vi "lockin - replace AO Sweep Indicator.vi"(8 "error in (no error)":errorcluster, 10 "Channels: AO.Sweep?":bool[](array[boolean]), 11 "LockinDAQ":refnum<class "LockinDAQ.lvclass">) -> (0 "error out":errorcluster, 3 "LockinDAQ out":refnum<class "LockinDAQ.lvclass">)   [LabVIEW 2019, in "LockinDAQ.lvclass"]
uses:
  LockinDAQ.lvclass
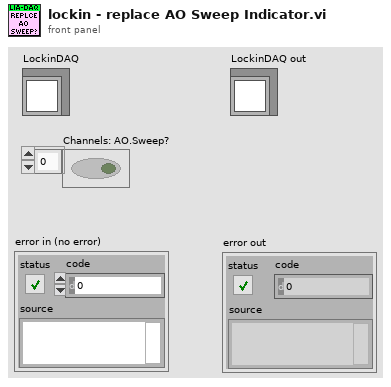
[diagram p1: front panel]
types:
  T1 = typedef "LockinDAQ.lvclass/AO-cluster.ctl" = cluster{"Ch":i32[], "Amp (V)":dbl[], "DC (V)":dbl[], "f (Hz)":dbl[], "Phase (°)":dbl[], "Function":T2[], "Sweep?":bool[]}
  T2 = typedef "LockinDAQ.lvclass/Function-enum.ctl" = enum16{"Sine", "Triangle", "Square", "Sawtooth"}
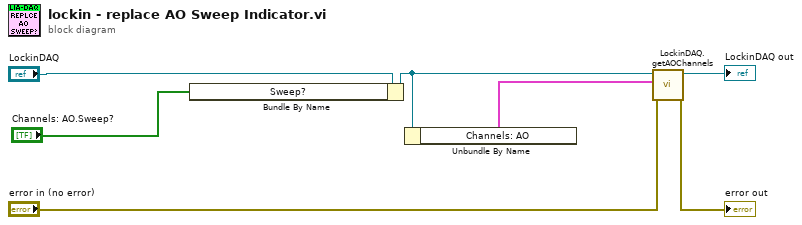
[diagram p0: block diagram]
diagram:
  n1 = Bundle By Name(cluster="LockinDAQ", "Sweep?"="Channels: AO.Sweep?") -> (w5:refnum<class "LockinDAQ.lvclass">)
  n2 = Unbundle By Name(w5) -> ("Channels: AO"=w6:T1)
  n3 = call "LockinDAQ.getAOChannels.vi"("error in (no error)"="error in (no error)", "Channels: AO"=w6, "LockinDAQ"=w5) -> ("error out"=→"error out":errorcluster, "LockinDAQ out"=→"LockinDAQ out":refnum<class "LockinDAQ.lvclass">)  [unwired: 7 in]
